vi "SetVISAResourceName.vi"(0 "object in":refnum<class "Valve.lvclass">, 1 "VISA resource name":refnum<visa-resource-name>, 5 "error in (no error)":errorcluster) -> (14 "object out":refnum<class "Valve.lvclass">, 19 "error out":errorcluster)   [LabVIEW 2019, in "Valve.lvclass"]
uses:
  Valve.lvclass
  Valve.lvclass/Valve.ctl
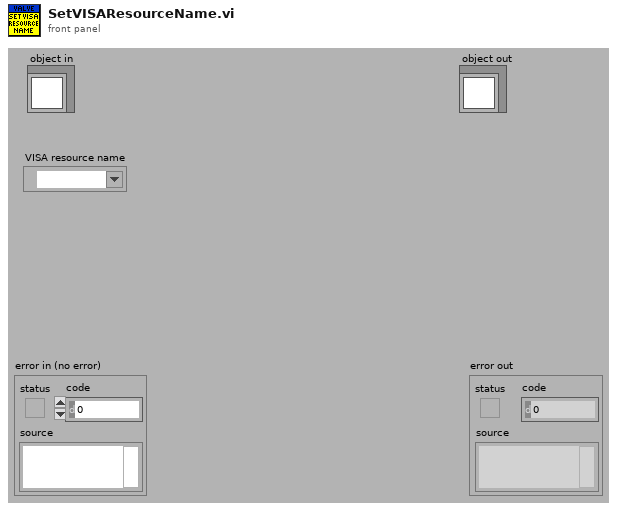
[diagram p1: front panel]
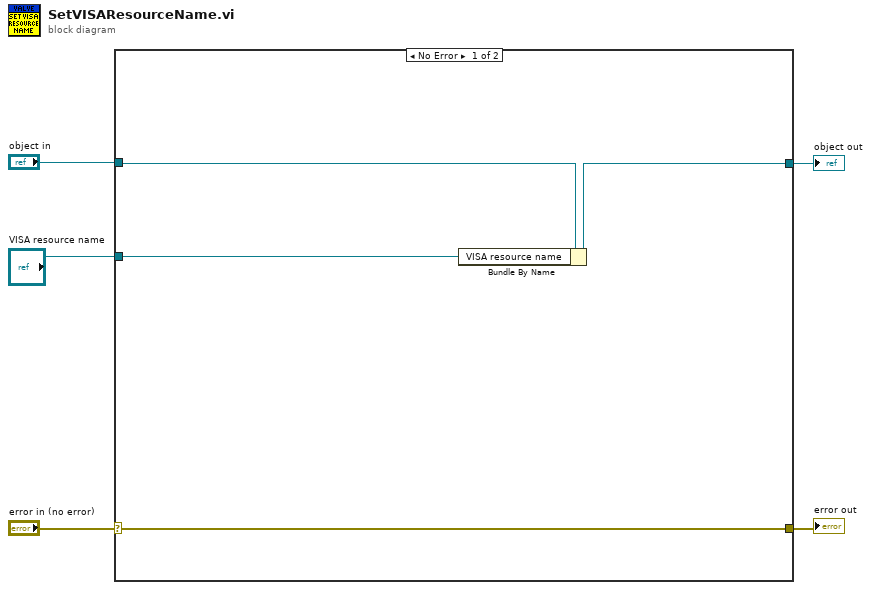
[diagram p0: block diagram]
diagram:
  n1 = case shown="No Error" "error in (no error)" {
    selector: "error in (no error)" -> [w8 w11]
    tunnel: [w8 w11] -> w4
    tunnel: [w6 w10] -> w2
    tunnel: "object in" -> [w7 w10]
    tunnel: "VISA resource name" -> [w9 _]
    frame No Error {
      n2 = Bundle By Name(cluster=w7, "VISA resource name"=w9) -> (w6:refnum<class "Valve.lvclass">)
    }
    frame Error {
    }
  }
  "error out" <- w4
  "object out" <- w2
